vi "TOOL-Cal arrays concatenation.vi"() -> ()   [LabVIEW 2017]
panel:
  out "appended array":dbl[][](array[numeric])
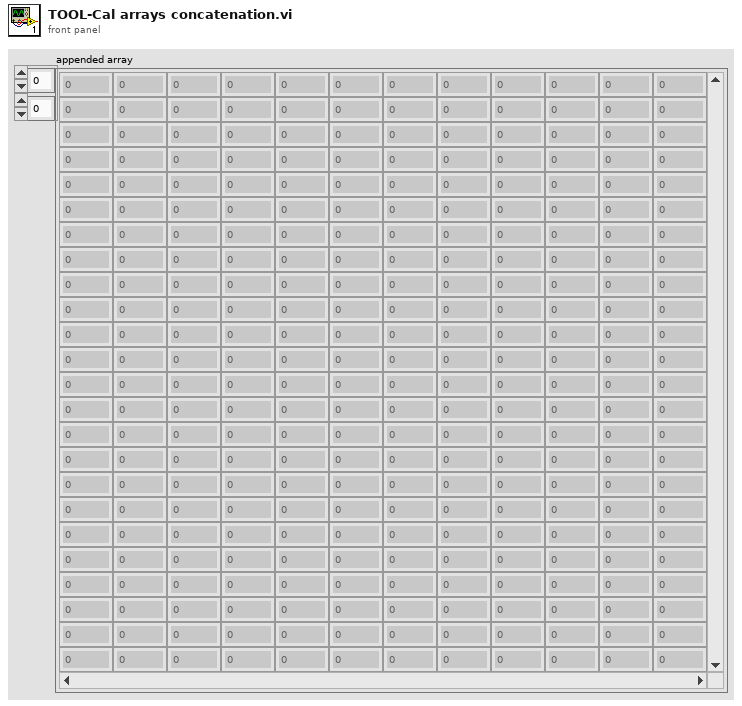
[diagram p1: front panel]
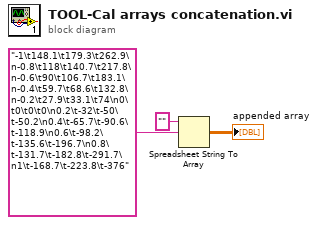
[diagram p0: block diagram]
diagram:
  n1 = Spreadsheet String To Array(format string="", spreadsheet string="-1\t148.1\t179.3\t262.9\n-0.8\t118\t140.7\t217.8\n-0.6\t90\t106.7\t183.1\n-0.4\t59.7\t68.6\t132.8\n-0.2\t27.9\t33.1\t74\n0\t0\t0\t0\n0.2\t-32\t-50\t-50.2\n0.4\t-65.7\t-90.6\t-118.9\n0.6\t-98.2\t-135.6\t-196.7\n0.8\t-131.7\t-182.8\t-291.7\n1\t-168.7\t-223.8\t-376") -> (array=→"appended array":dbl[][])  [unwired: 2 in]
